vi "P02_Filtro Feedback Node Emma 2.vi"() -> ()   [LabVIEW 2026]
panel:
  in  "stop":bool
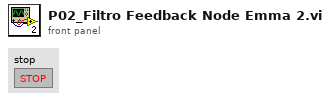
[diagram p1: front panel]
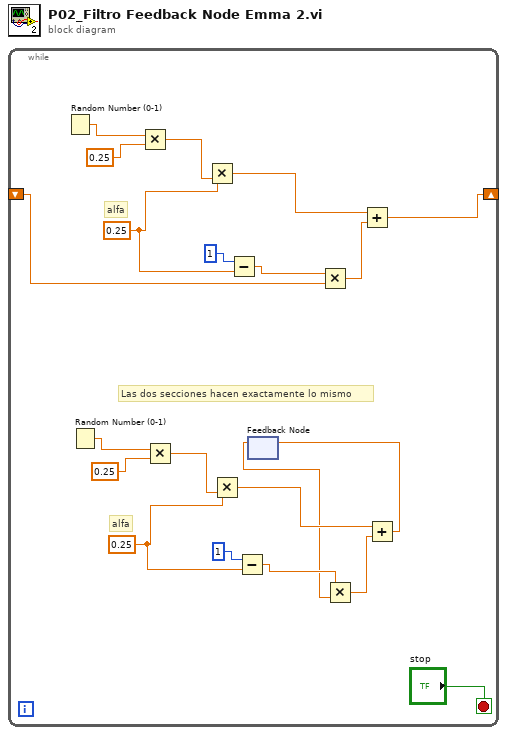
[diagram p0: block diagram]
diagram:
  n1 = while {
    shift-right: [w15] -> _
    shift-left: _ -> [w12]
    stop <- "stop" stop-if-true
    w6 = 0.25
    w17 = 0.25
    # "Las dos secciones hacen exactamente lo mismo"
    # "alfa"
    # "alfa"
    n2 = Random Number (0-1)() -> (number: 0 to 1=w20:dbl)
    n3 = Random Number (0-1)() -> (number: 0 to 1=w9:dbl)
    n4 = Multiply(x=w20, y=0.25) -> (x*y=w19:dbl)
    n5 = Multiply(x=w9, y=0.25) -> (x*y=w8:dbl)
    n6 = Multiply(x=w17, y=w19) -> (x*y=w16:dbl)
    n7 = Multiply(x=w6, y=w8) -> (x*y=w5:dbl)
    n8 = Subtract(x=1, y=w17) -> (x-y=w13:dbl)
    n9 = Subtract(x=1, y=w6) -> (x-y=w4:dbl)
    n10 = feedback #1() -> (w1:dbl)  [unwired: 1 in]
    n11 = Multiply(x=w13, y=w12) -> (x*y=w11:dbl)
    n12 = Multiply(x=w4, y=w1) -> (x*y=w3:dbl)
    n13 = Add(x=w16, y=w11) -> (x+y=w15:dbl)
    n14 = Add(x=w5, y=w3) -> (x+y=w2:dbl)
    n15 = feedback-in #1(w2) -> ()
  }
